vi "Set Device DTR.vi"(8 "error in (no error)":errorcluster, 11 "Handle":u64) -> (0 "error out":errorcluster, 3 "Handle out":u64)   [LabVIEW 2019, in "D2XX-lv.lvlib"]
doc: "This function sets the Data Terminal Ready (DTR) control signal of an open device."
uses:
  D2XX-lv.lvlib
  <instrlib>/_D2XX/D2XX/D2XX.lvlib
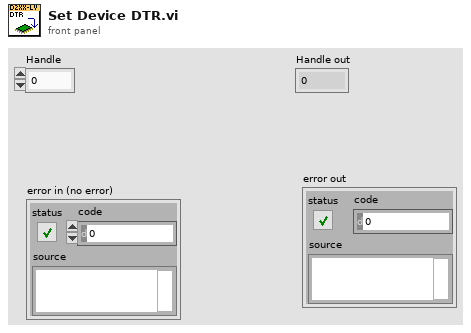
[diagram p1: front panel]
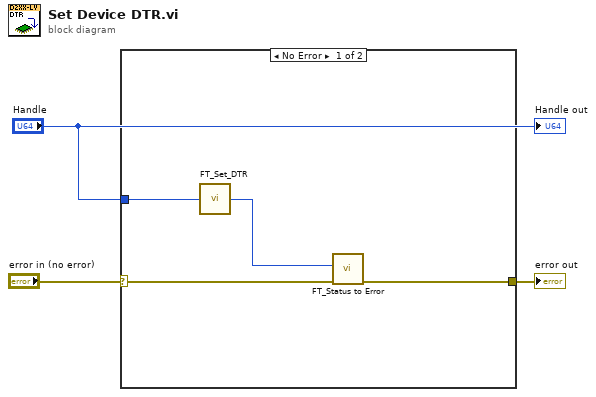
[diagram p0: block diagram]
diagram:
  n1 = case shown="No Error" "error in (no error)" {
    selector: "error in (no error)" -> [w7 w8]
    tunnel: [w4 w8] -> w2
    tunnel: "Handle" -> [w6 _]
    frame No Error {
      n2 = call <instrlib>:"FT_Set_DTR.vi"("Handle"=w6) -> ("FT_Status"=w5:u32)
      n3 = call "FT_Status to Error.vi"("error in (no error)"=w7, "FT_Status"=w5) -> ("error out"=w4:errorcluster)  [unwired: 9 in]
    }
    frame Error {
    }
  }
  "error out" <- w2
  "Handle out" <- "Handle"
